vi "setAttributeTreeValue.vi"(0 "HGF_IMAQDevice":refnum<class "HGF_IMAQDevice.lvclass">, 1 "Tree Control In":refnum<vi>, 3 "Tab Control Ref In":T1, 5 "error in (no error)":errorcluster) -> (14 "dup HGF_IMAQDevice":refnum<class "HGF_IMAQDevice.lvclass">, 15 "Tree Control Out":refnum<vi>, 19 "error out":errorcluster)   [LabVIEW 2014, in "HGF_IMAQ.lvlib" / "HGF_IMAQDevice.lvclass"]
doc: "This is the override VI to set cameras selected attribute value."
uses:
  HGF_IMAQDevice.lvclass
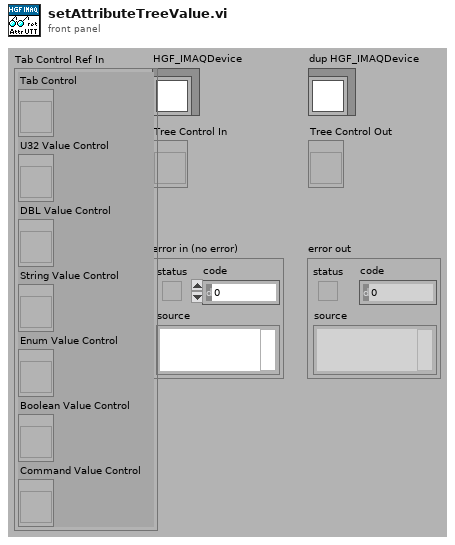
[diagram p1: front panel]
types:
  T1 = cluster{"Tab Control":refnum<vi>, "U32 Value Control":refnum<vi>, "DBL Value Control":refnum<vi>, "String Value Control":refnum<vi>, "Enum Value Control":refnum<vi>, "Boolean Value Control":refnum<vi>, "Command Value Control":refnum<vi>}
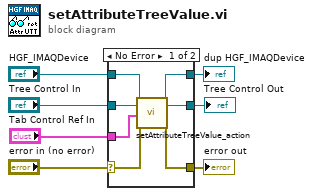
[diagram p0: block diagram]
diagram:
  n1 = case shown="No Error" "error in (no error)" {
    selector: "error in (no error)" -> [w14 w15]
    tunnel: [w13 w15] -> w6
    tunnel: [w10 w16] -> w4
    tunnel: "HGF_IMAQDevice" -> [w11 w16]
    tunnel: "Tree Control In" -> [w12 _]
    tunnel: [w9 _] -> w2
    tunnel: "Tab Control Ref In" -> [w8 _]
    frame No Error {
      n2 = call-dynamic "setAttributeTreeValue_action.vi"("HGF_IMAQDevice"=w11, "Tree Control In"=w12, "Tab Control Ref In"=w8, "error in (no error)"=w14) -> ("dup HGF_IMAQDevice"=w10:refnum<class "HGF_IMAQDevice.lvclass">, "Tree Control Out"=w9:refnum<vi>, "error out"=w13:errorcluster)  [unwired: 13 in]
    }
    frame Error {
    }
  }
  "error out" <- w6
  "dup HGF_IMAQDevice" <- w4
  "Tree Control Out" <- w2
